vi "SerialJudge.vi"() -> ()   [LabVIEW 2013]
panel:
  in  "128K？":bool
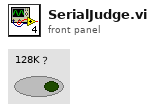
[diagram p1: front panel]
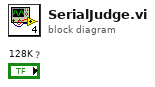
[diagram p0: block diagram]
diagram:
